vi "题目4.vi"() -> ()   [LabVIEW 2017]
panel:
  in  "枚举":enum16{"张三", "李四", "王五"}(ring)
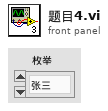
[diagram p1: front panel]
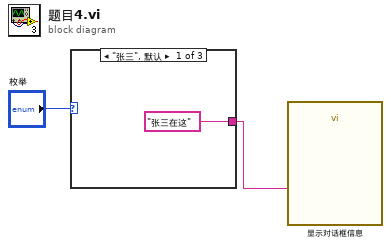
[diagram p0: block diagram]
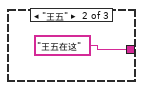
[diagram p2: hidden frame]
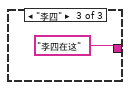
[diagram p3: hidden frame]
diagram:
  n1 = case shown="\"张三\", 默认" "枚举" {
    tunnel: ["张三在这" "王五在这" "李四在这"] -> w1
    frame "张三", Default {
    }
    frame "王五" {
    }
    frame "李四" {
    }
  }
  n2 = call "显示对话框信息"("Message"=w1) -> ()  [unwired: 9 in, 2 out]
